vi "niRFUtil RFHS Filter Info.vi"(0 "Channelizer Spec":T4={"freq in Hz"=TRUE, "Filter Type Hint"=enum."Auto", "Hint Value"=0.0, "Channels"=[]} {"Channels"."Flags" items=["None"=0, "Force Fractional"=1, "Use Multistage"=2, "Use Pretrigger Data "=256, "Frequency Shift Only"=4]; "Channels"."fs" format="%#_8p"; "Channels"."fc" format="%#_6p"; "Channels"."stopBW" format="%#_6p"; "Channels"."passBW" format="%#_6p"; "Hint Value" format="%#_8p"}, 1 "Filter Purpose":T2, 5 "fs [Hz]":dbl=1000000000.0 format="%#_6p", 7 "#input samples":dbl, 9 "#output samples":dbl, 11 "error in (no error)":errorcluster) -> (4 "Stage Info":T3[](array[typedef]), 6 "Pre/Post Trigger Filter Info":T1, 8 "#output samples (#input samples)":dbl, 10 "#input samples (#output samples)":dbl, 15 "error out":errorcluster)   [LabVIEW 2015, in "niRFUtil.lvlib"]
uses:
  niRFUtil.lvlib
  Includes/niRFUtil RFHS Channelizer ChannelSpecification.ctl
  Includes/niRFUtil RFHS Channelizer FilterTypeHint.ctl
  Includes/niRFUtil RFHS Channelizer ChannelSpecificationBase.ctl
  Includes/niRFUtil RFHS Channelizer ChannelFlags.ctl
  Includes/niRFUtil RFHS Filter Info.ctl
  Includes/niRFUtil RFHS Channelizer FilterPurpose.ctl
  Includes/niRFUtil RFHS Filter Pre Post Trigger Info.ctl
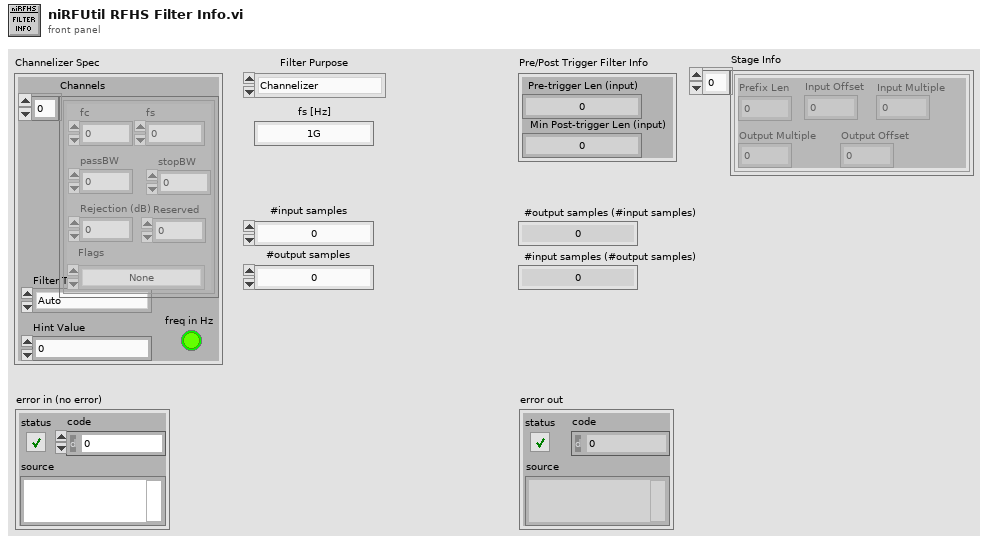
[diagram p1: front panel]
types:
  T1 = typedef "niRFUtil.lvlib/niRFUtil RFHS Filter Pre Post Trigger Info.ctl" = cluster{"Pre-trigger Len (input)":i64, "Min Post-trigger Len (input)":i64}
  T2 = typedef "niRFUtil.lvlib/niRFUtil RFHS Channelizer FilterPurpose.ctl" = enum16{"Channelizer", "Fine Tune Resampler"}
  T3 = typedef "niRFUtil.lvlib/niRFUtil RFHS Filter Info.ctl" = cluster{"Prefix Len":i32, "Input Offset":i32, "Input Multiple":i32, "Output Multiple":dbl, "Output Offset":i32}
  T4 = typedef "niRFUtil.lvlib/niRFUtil RFHS Channelizer ChannelSpecification.ctl" = cluster{"freq in Hz":bool, "Filter Type Hint":T5, "Hint Value":dbl, "Channels":T6[]}
  T5 = typedef "niRFUtil.lvlib/niRFUtil RFHS Channelizer FilterTypeHint.ctl" = enum16{"Auto", "FFT (LTE)", "FFT (WiFi)", "FFT (custom)"}
  T6 = typedef "niRFUtil.lvlib/niRFUtil RFHS Channelizer ChannelSpecificationBase.ctl" = cluster{"fc":dbl, "fs":dbl, "passBW":dbl, "stopBW":dbl, "Rejection (dB)":dbl, "Flags":T7, "Reserved":i32}
  T7 = typedef "niRFUtil.lvlib/niRFUtil RFHS Channelizer ChannelFlags.ctl" = u32
  T8 = typedef "niRFUtil.lvlib/niRFUtil RFHS Channelizer FilterSpecification.ctl" = cluster{"Type":enum32{"Reserved", "Rational", "Fine Tune", "Fractional", "Rational (user)", "Reserved 2", "Fractional (user)", "FFT Resampler"}, "Reserved":i32, "Spec":T6}
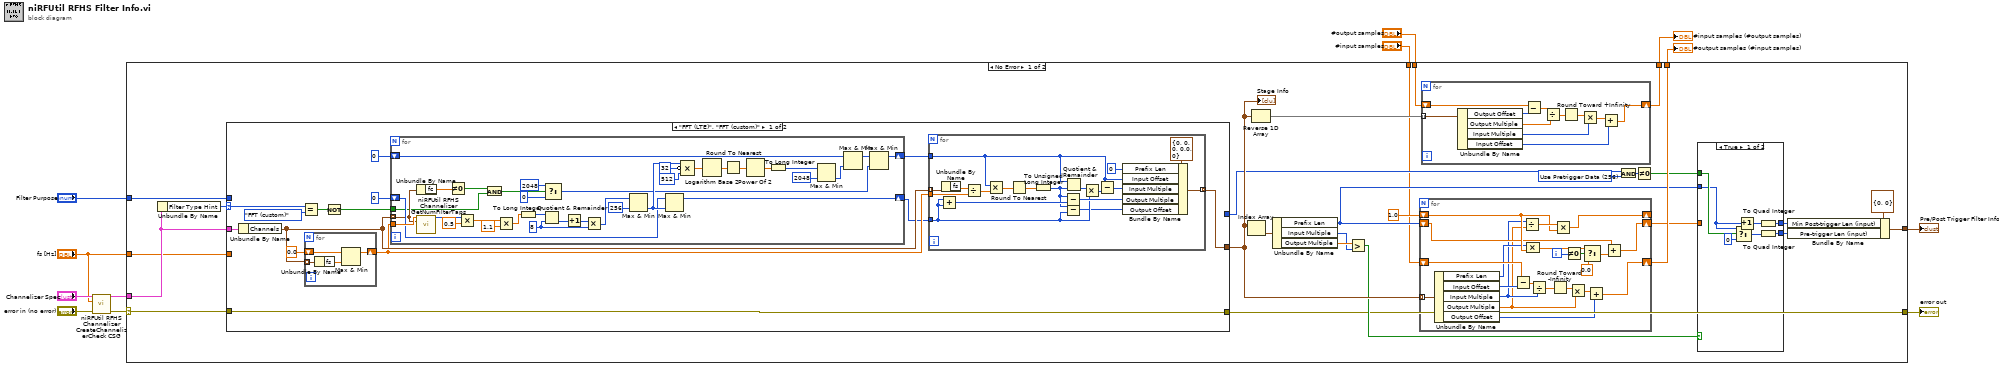
[diagram p0: block diagram]
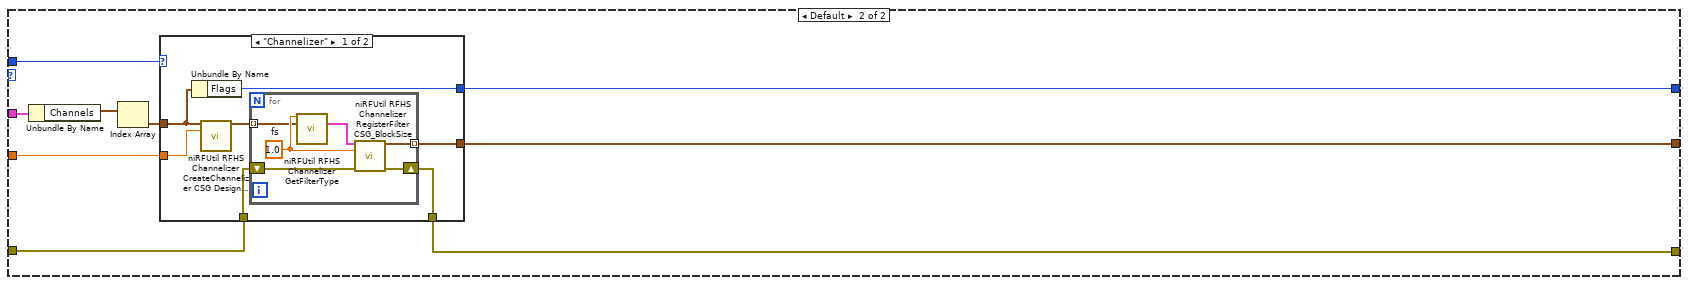
[diagram p2: hidden frame]
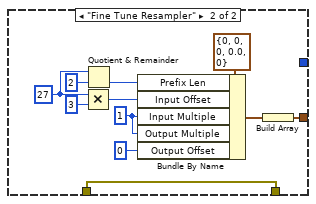
[diagram p3: hidden frame]
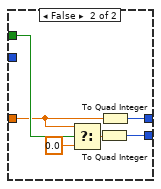
[diagram p4: hidden frame]
diagram:
  n1 = call "niRFUtil RFHS Channelizer CreateChannelizerCheck CSG.vi"("Channel Spec"="Channelizer Spec", "fs [Hz]"="fs [Hz]", "error in (no error)"="error in (no error)") -> ("Channel Spec (out)"=w11:T4, "error out"=w4:errorcluster)  [unwired: 11 in]
  n2 = case shown="No Error" w4 {
    selector: w4 -> [w20 w190]
    tunnel: w11 -> [w39 _]
    tunnel: "Filter Purpose" -> [w38 _]
    tunnel: "fs [Hz]" -> [w37 _]
    tunnel: [w35 _] -> w7
    tunnel: [w34 _] -> w6
    tunnel: [w19 _] -> w5
    tunnel: [w15 w190] -> w3
    tunnel: "#output samples" -> [w14 _]
    tunnel: "#input samples" -> [w13 _]
    frame No Error {
      w29 = T7 256 items=["None"=0, "Force Fractional"=1, "Use Multistage"=2, "Use Pretrigger Data "=256] ("y")
      n3 = Unbundle By Name(w39) -> ("Filter Type Hint"=w21:T5)
      n4 = case shown="\"FFT (LTE)\", \"FFT (custom)\"" w21 {
        selector: w21 -> [w45 _]
        tunnel: w39 -> [w53 w118]
        tunnel: [w41 w113] -> w31
        tunnel: w38 -> [_ w116]
        tunnel: w20 -> [w40 w115]
        tunnel: [w40 w114] -> w15
        tunnel: w37 -> [_ w112]
        tunnel: [_ w111] -> w30
        frame "FFT (LTE)", "FFT (custom)" {
          n5 = Unbundle By Name(w53) -> ("Channels"=w50:T6[])
          n6 = Equal?(x=w45, y=niRFUtil_RFHS_Channelizer_FilterTypeHint."FFT (custom)") -> (x = y?=w44:bool)
          n7 = for {
            tunnel: w50 -> [w75] mode=indexing
            shift-right: [w73] -> w49
            shift-left: 0.0 -> [w72]
            n8 = Unbundle By Name(w75) -> ("fs"=w74:dbl)
            n9 = Max & Min(x=w72, y=w74) -> (max(x,y)=w73:dbl)  [unwired: 1 out]
          }
          n10 = Not(x=w44) -> (.not. x?=w43:bool)
          n11 = for {
            tunnel: w50 -> [w85] mode=indexing
            shift-right: [w76] -> w47
            shift-left: 0 -> [w92]
            tunnel: w49 -> [w91]
            shift-right: [w87] -> w42
            shift-left: 0 -> [w88]
            tunnel: w43 -> [w82]
            w101 = 8 ("y")
            n12 = Unbundle By Name(w85) -> ("fc"=w84:dbl)
            n13 = call "niRFUtil RFHS Channelizer GetNumFilterTaps.vi"("fs"=w91, "Channel Specification"=w85) -> ("#Filter Taps"=w90:i32)  [unwired: 13 in]
            n14 = Not Equal To 0?(x=w84) -> (x != 0?=w83:bool)
            n15 = Multiply(x=w90, y=0.5) -> (x*y=w94:dbl)
            n16 = And(x=w83, y=w82) -> (x .and. y?=w80:bool)
            n17 = Multiply(x=w94, y=1.1) -> (x*y=w96:dbl)
            n18 = To Long Integer(number=w96) -> (32bit integer=w98:i32)
            n19 = Quotient & Remainder(x=w98, y=w101) -> (floor(x/y)=w99:i32)  [unwired: 1 out]
            n20 = Select(t=2048 ("Len Hint"), s=w80, f=0 ("Len Hint")) -> (s? t:f=w77:i32)
            n21 = Increment(x=w99) -> (x+1=w100:i32)
            n22 = Multiply(x=w100, y=w101) -> (x*y=w102:i32)
            n23 = Max & Min(x=w102, y=256) -> (min(x,y)=w89:i32)  [unwired: 1 out]
            n24 = Max & Min(x=w88, y=w89) -> (max(x,y)=w87:i32)  [unwired: 1 out]
            n25 = Compound Arithmetic op=MULTIPLY(w89, invert 32 ("value"), 512 ("value")) -> (w105:dbl)
            n26 = Logarithm Base 2(1:w105) -> (0:w106:dbl)
            n27 = Round To Nearest(number=w106) -> (nearest integer value=w107:dbl)
            n28 = Power Of 2(x=w107) -> (2^x=w108:dbl)
            n29 = To Long Integer(number=w108) -> (32bit integer=w109:i32)
            n30 = Max & Min(x=w109, y=2048) -> (min(x,y)=w86:i32)  [unwired: 1 out]
            n31 = Max & Min(x=w92, y=w86) -> (max(x,y)=w78:i32)  [unwired: 1 out]
            n32 = Max & Min(x=w78, y=w77) -> (max(x,y)=w76:i32)  [unwired: 1 out]
          }
          n33 = for {
            tunnel: w50 -> [w71] mode=indexing
            tunnel: w47 -> [w63]
            tunnel: w49 -> [w67]
            tunnel: w42 -> [w56]
            tunnel: [w54] -> w41 mode=indexing
            n34 = Add(x=w56, y=w56) -> (x+y=w59:i32)
            n35 = Unbundle By Name(w71) -> ("fs"=w68:dbl)
            n36 = Divide(x=w68, y=w67) -> (x/y=w66:dbl)
            n37 = Multiply(x=w63, y=w66) -> (x*y=w70:dbl)
            n38 = Round To Nearest(number=w70) -> (nearest integer value=w69:dbl)
            n39 = To Unsigned Long Integer(number=w69) -> (unsigned 32bit integer=w57:u32)
            n40 = Subtract(x=w57, y=w59) -> (x-y=w58:u32)
            n41 = Subtract(x=w57, y=w56) -> (x-y=w55:u32)
            n42 = Quotient & Remainder(x=w63, y=w57) -> (floor(x/y)=w62:u32)  [unwired: 1 out]
            n43 = Multiply(x=w62, y=w56) -> (x*y=w61:u32)
            n44 = Subtract(x=w63, y=w61) -> (x-y=w60:u32)
            n45 = Bundle By Name(cluster=T3 {"Prefix Len"=0, "Input Offset"=0, "Input Multiple"=0, "Output Multiple"=0.0, "Output Offset"=0} ("Filter Info"), "Prefix Len"=0, "Input Offset"=w63, "Input Multiple"=w60, "Output Multiple"=w58, "Output Offset"=w55) -> (w54:T3)
          }
        }
        frame Default {
          n46 = Unbundle By Name(w118) -> ("Channels"=w119:T6[])
          n47 = Index Array(array=w119) -> (element=w117:T6)  [unwired: 1 in]
          n48 = case shown="\"Channelizer\"" w116 {
            tunnel: w117 -> [w121 _]
            tunnel: [w124 w133] -> w113
            tunnel: w115 -> [w126 w134]
            tunnel: [w125 w134] -> w114
            tunnel: w112 -> [w123 _]
            tunnel: [w120 _] -> w111
            frame "Channelizer" {
              n49 = Unbundle By Name(w121) -> ("Flags"=w120:T7)
              n50 = call "niRFUtil RFHS Channelizer CreateChannelizer CSG Design Stages.vi"("Channel Spec"=w121, "fs"=w123) -> ("Stages"=w122:T6[])  [unwired: 11 in, 2 out]
              n51 = for {
                shift-right: [w131] -> w125
                shift-left: w126 -> [w132]
                tunnel: [w128] -> w124 mode=indexing
                tunnel: w122 -> [w127] mode=indexing
                w129 = 1.0  # fs
                n52 = call "niRFUtil RFHS Channelizer GetFilterType.vi"("fs"=w129, "Channel Specification"=w127) -> ("Filter Spec"=w130:T8)  [unwired: 10 in, 3 out]
                n53 = call "niRFUtil RFHS Channelizer RegisterFilter CSG_BlockSize.vi"("Filter Spec"=w130, "fs"=w129, "error in (no error)"=w132) -> ("Filter Info"=w128:T3, "error out"=w131:errorcluster)  [unwired: 11 in]
              }
            }
            frame "Fine Tune Resampler" {
              w136 = 27 ("y")
              w138 = 1 ("Input Multiple")
              n54 = Multiply(x=w136, y=3) -> (x*y=w139:i32)
              n55 = Quotient & Remainder(x=w136, y=2) -> (floor(x/y)=w141:i32)  [unwired: 1 out]
              n56 = Bundle By Name(cluster=T3 {"Prefix Len"=0, "Input Offset"=0, "Input Multiple"=0, "Output Multiple"=0.0, "Output Offset"=0} ("Filter Info 2"), "Prefix Len"=w141, "Input Offset"=w139, "Input Multiple"=w138, "Output Multiple"=w138, "Output Offset"=0) -> (w135:T3)
              n57 = Build Array(w135) -> (w133:T3[])
            }
          }
        }
      }
      "Stage Info" <- w31
      n58 = Index Array(array=w31) -> (element=w32:T3)  [unwired: 1 in]
      n59 = Reverse 1D Array(array=w31) -> (reversed array=w36:T3[])
      n60 = Unbundle By Name(w32) -> ("Prefix Len"=w24:i32, "Input Multiple"=w26:i32, "Output Multiple"=w27:dbl)
      n61 = Greater?(x=w27, y=w26) -> (0:w25:bool)
      n62 = for {
        tunnel: w31 -> [w162] mode=indexing
        shift-right: [w173] -> w34
        shift-left: w13 -> [w174]
        shift-right: [w171] -> _
        shift-left: 1.0 -> [w170]
        shift-right: [w164] -> w28
        shift-left: w24 -> [w163]
        i -> [w168]
        n63 = Unbundle By Name(w162) -> ("Prefix Len"=w159:i32, "Input Offset"=w160:i32, "Input Multiple"=w158:i32, "Output Multiple"=w157:dbl, "Output Offset"=w161:i32)
        n64 = Subtract(x=w174, y=w160) -> (x-y=w178:dbl)
        n65 = Divide(x=w158, y=w157) -> (x/y=w172:dbl)
        n66 = Compound Arithmetic op=MULTIPLY(w159, w170) -> (w166:dbl)
        n67 = Divide(x=w178, y=w158) -> (x/y=w177:dbl)
        n68 = Round Toward -Infinity(1:w177) -> (0:w176:dbl)
        n69 = Multiply(x=w172, y=w170) -> (x*y=w171:dbl)
        n70 = Not Equal To 0?(x=w168) -> (x != 0?=w169:bool)
        n71 = Multiply(x=w176, y=w157) -> (x*y=w175:dbl)
        n72 = Select(t=w166, s=w169, f=0.0) -> (s? t:f=w165:dbl)
        n73 = Add(x=w175, y=w161) -> (x+y=w173:dbl)
        n74 = Add(x=w163, y=w165) -> (x+y=w164:dbl)
      }
      n75 = for {
        tunnel: w36 -> [w183] mode=indexing
        shift-right: [w184] -> w35
        shift-left: w14 -> [w185]
        n76 = Unbundle By Name(w183) -> ("Output Offset"=w179:i32, "Output Multiple"=w180:dbl, "Input Multiple"=w181:i32, "Input Offset"=w182:i32)
        n77 = Subtract(x=w185, y=w179) -> (x-y=w189:dbl)
        n78 = Divide(x=w189, y=w180) -> (x/y=w188:dbl)
        n79 = Round Toward +Infinity(x=w188) -> (ceil(x): smallest int >= x=w187:dbl)
        n80 = Multiply(x=w187, y=w181) -> (x*y=w186:dbl)
        n81 = Add(x=w186, y=w182) -> (x+y=w184:dbl)
      }
      n82 = And(x=w30, y=w29) -> (x .and. y?=w23:T7)
      n83 = Not Equal To 0?(x=w23) -> (x != 0?=w22:bool)
      n84 = case shown="True" w25 {
        tunnel: w28 -> [_ w154]
        tunnel: w24 -> [w148 _]
        tunnel: w22 -> [w150 w155]
        tunnel: [w145 w152] -> w17
        tunnel: [w144 w151] -> w16
        frame True {
          n85 = Select(t=w148, s=w150, f=0) -> (s? t:f=w146:i32)
          n86 = Increment(x=w148) -> (x+1=w147:i32)
          n87 = To Quad Integer(1:w147) -> (0:w145:i64)
          n88 = To Quad Integer(1:w146) -> (0:w144:i64)
        }
        frame False {
          n89 = Select(t=w154, s=w155, f=0.0) -> (s? t:f=w153:dbl)
          n90 = To Quad Integer(1:w153) -> (0:w151:i64)
          n91 = To Quad Integer(1:w154) -> (0:w152:i64)
        }
      }
      n92 = Bundle By Name(cluster=T1 {"Pre-trigger Len (input)"=0, "Min Post-trigger Len (input)"=0} ("Pre/Post Trigger Filter Info"), "Min Post-trigger Len (input)"=w17, "Pre-trigger Len (input)"=w16) -> (w19:T1)
    }
    frame Error {
    }
  }
  "#input samples (#output samples)" <- w7
  "#output samples (#input samples)" <- w6
  "Pre/Post Trigger Filter Info" <- w5
  "error out" <- w3
